vi "_io_read_long_data.vi"(4 "Simulation read buffer (\"Simulation\")":string="Simulation", 6 "Block Logging (F)":bool, 7 "Block Delay Before Read (F)":bool, 8 "error in":errorcluster caption="error in (no error)", 9 "Trim Response End (T)":bool=TRUE, 10 "Max segment read bytes count (65536)":u32=65536, 11 "VISA resource name":refnum<visa-resource-name>) -> (0 "error out":errorcluster, 1 "Read bytes count":u32, 2 "Read buffer":string, 3 "VISA resource name out":refnum<visa-resource-name>)   [LabVIEW 2022 SP3, in "hmp4000_rsidr_core.lvlib"]
uses:
  hmp4000_rsidr_core.lvlib
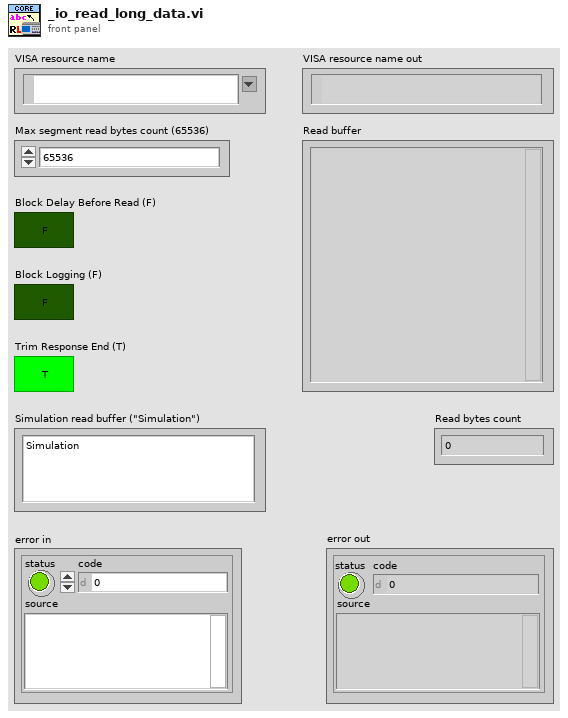
[diagram p1: front panel]
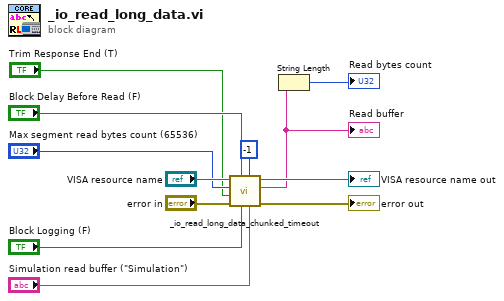
[diagram p0: block diagram]
diagram:
  n1 = call "_io_read_long_data_chunked_timeout.vi"("Simulation read buffer (\"Simulation\")"="Simulation read buffer (\"Simulation\")", "Timeout for chunked touts (-1: No chunked touts)"=-1, "Block Logging (F)"="Block Logging (F)", "Block Delay Before Read (F)"="Block Delay Before Read (F)", "error in"="error in", "Trim Response End"="Trim Response End (T)", "Max segment read bytes count (65536)"="Max segment read bytes count (65536)", "VISA resource name"="VISA resource name") -> ("error out"=→"error out":errorcluster, "Read buffer"=w2:string, "VISA resource name out"=→"VISA resource name out":refnum<visa-resource-name>)  [unwired: 1 out]
  "Read buffer" <- w2
  n2 = String Length(string=w2) -> (length=→"Read bytes count":i32)
